vi "_Construct CellValue.vi"(8 "error in":errorcluster, 11 "Text":string) -> (0 "error out":errorcluster, 3 "CellValue out":refnum<k24>)   [LabVIEW 2021, in "Open Xml.lvlib"]
uses:
  Open Xml.lvlib
  D:/git/Open-Xml-LabVIEW/dll/DocumentFormat.OpenXml.dll
  dll/DocumentFormat.OpenXml.dll
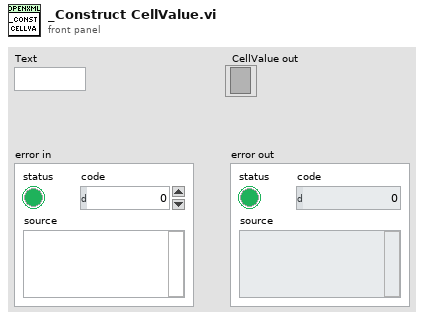
[diagram p1: front panel]
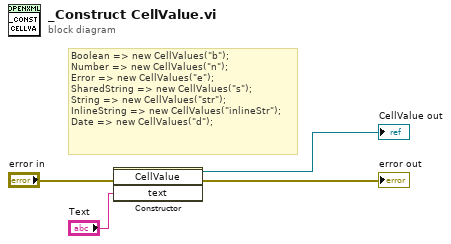
[diagram p0: block diagram]
diagram:
  # "Boolean => new CellValues(\"b\");\nNumber => new CellValues(\"n\");\nError => new CellValues(\"e\");\nSharedString => new CellValues(\"s\");\nString => new CellValues(\"str\");\nInlineString => new CellValues(\"inlineStr\");\nDate => new CellValues(\"d\");"
  n1 = constructor class="CellValue"(error in="error in", "text"="Text") -> (reference out=→"CellValue out":refnum<k24>, error out=→"error out":errorcluster)  [unwired: 2 in, 2 out]
